vi "SGDA-Initialize Hardware.vi"(0 "Start PXI Server":bool=TRUE, 7 "TDT-Device Config":T1, 11 "error in (no error)":errorcluster) -> (8 "Hardware":T5, 15 "error out":errorcluster)   [LabVIEW 2020]
uses:
  Type Defs/Hardware Destination.ctl
  TDT VIs/Typedefs/TDT-Device Config.ctl
  TDT VIs/Typedefs/TDT-Output source.ctl
  TDT VIs/Typedefs/TDT-Device ID.ctl
  TDT VIs/Typedefs/TDT-Input source.ctl
  SGDA-Globals.vi
  <resource>/objmgr/daqmx.rc
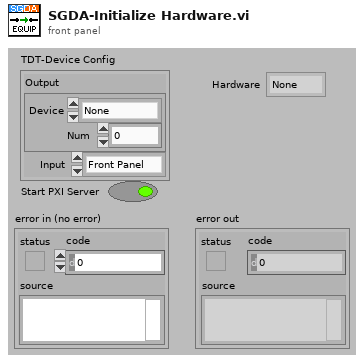
[diagram p1: front panel]
types:
  T1 = typedef "TDT-Device Config.ctl" = cluster{"Output":T2, "Input":T4}
  T2 = typedef "TDT-Output source.ctl" = cluster{"Device":T3, "Num":i32}
  T3 = typedef "TDT-Device ID.ctl" = enum16{"None", "PA5", "RP2", "RL2", "RA16", "RV8", "RX5", "RX6", "RX7", "RX8", "RZ2", "RZ5", "RZ6"}
  T4 = typedef "TDT-Input source.ctl" = enum16{"Front Panel", "RA4LI", "RA16LI"}
  T5 = typedef "Hardware Destination.ctl" = enum16{"None", "PXI", "TDT", "NI", "TDTSIM"}
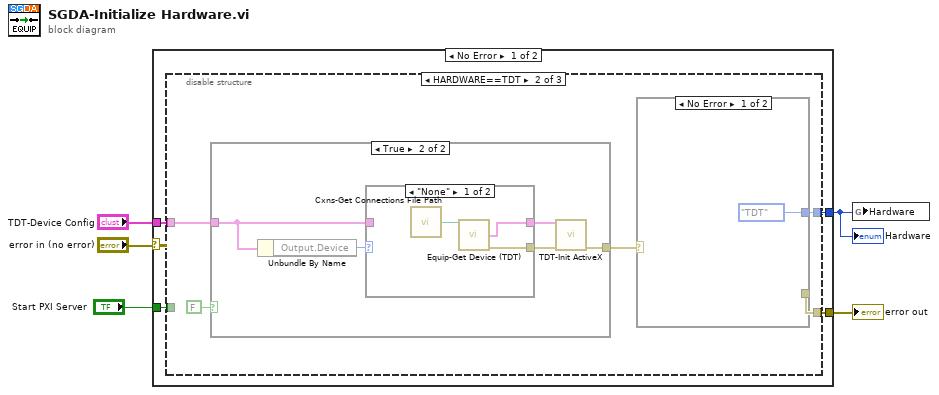
[diagram p0: block diagram]
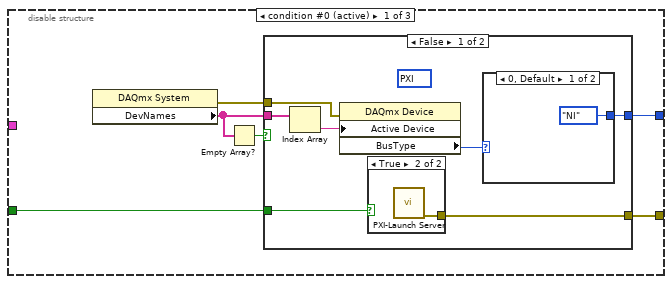
[diagram p2: hidden frame]
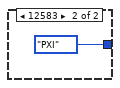
[diagram p4: hidden frame]
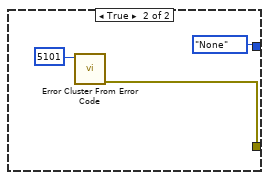
[diagram p5: hidden frame]
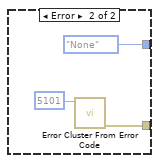
[diagram p8: hidden frame]
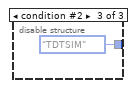
[diagram p9: hidden frame]
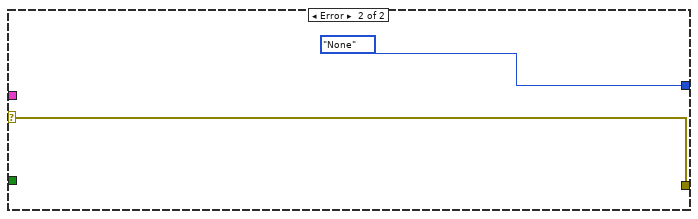
[diagram p10: hidden frame]
diagram:
  n1 = case shown="No Error" "error in (no error)" {
    selector: "error in (no error)" -> [_ w49]
    tunnel: [w9 w49] -> w4
    tunnel: [w8 Hardware_Destination."None" ("Hardware")] -> w3
    tunnel: "TDT-Device Config" -> [w7 _]
    tunnel: "Start PXI Server" -> [w6 _]
    frame No Error {
      n2 = disable-structure shown="HARDWARE==TDT" {
        disable-tunnel: [w15 w32 _] -> w9
        disable-tunnel: [w14 w31 Hardware_Destination."TDTSIM" ("Hardware")] -> w8
        disable-tunnel: w7 -> [_ w30 _]
        disable-tunnel: w6 -> [w13 _ _]
        frame condition #0 (active) {
          n3 = property class="DAQmx System"() -> (error out=w10:errorcluster, "DevNames"=w11:tag[])  [unwired: 2 in, 1 out]
          n4 = Empty Array?(array=w11) -> (empty?=w12:bool)
          n5 = case shown="False" w12 {
            tunnel: [w22 w27] -> w15
            tunnel: [w21 Hardware_Destination."None" ("Hardware")] -> w14
            tunnel: w11 -> [w20 _]
            tunnel: w10 -> [w18 _]
            tunnel: w13 -> [w16 _]
            frame False {
              (unwired) 12583 items=["PCI"=12582, "PCIe"=13612, "PXI"=12583, "PXIe"=14706, "SCXI"=12584, "SCC"=14707, "PCCard"=12585, "USB"=12586, "CompactDAQ"=14637, "TCP/IP"=14828, "Unknown"=12588, "SwitchBlock"=15870] ("BusType")
              n6 = Index Array(array=w20) -> (element=w19:tag)  [unwired: 1 in]
              n7 = property class="DAQmx Device"(error in=w18, "Active Device"=w19) -> ("BusType"=w17:i32)  [unwired: 1 in, 2 out]
              n8 = case shown="True" w16 {
                tunnel: [_ w23] -> w22
                frame False {
                }
                frame True {
                  n9 = call "PXI-Launch Server.vi"() -> ("error out"=w23:errorcluster)  [unwired: 10 in, 1 out]
                }
              }
              n10 = case shown="0, Default" w17 {
                tunnel: [Hardware_Destination."NI" ("Hardware") Hardware_Destination."PXI" ("Hardware")] -> w21
                frame 0, Default {
                }
                frame 12583 {
                }
              }
            }
            frame True {
              n11 = call <vilib>:"Error Cluster From Error Code.vi"("error code (0)"=5101) -> ("error out"=w27:errorcluster)  [unwired: 8 in]
            }
          }
        }
        frame condition #1 {
          n12 = case shown="True" FALSE {
            tunnel: [_ w38] -> w33
            tunnel: w30 -> [_ w36]
            frame False {
            }
            frame True {
              n13 = Unbundle By Name(w36) -> ("Output.Device"=w37:T3)
              n14 = case shown="\"None\"" w37 {
                tunnel: w36 -> [_ w42]
                tunnel: [w40 w42] -> w35
                tunnel: [w39 _] -> w34
                frame "None" {
                  n15 = call "Cxns-Get Connections File Path.vi"() -> ("Path Out"=w41:path)  [unwired: 1 in]
                  n16 = call "Equip-Get Device (TDT).vi"("Path In"=w41) -> ("TDT-Device Config"=w40:T1, "error out"=w39:errorcluster)  [unwired: 12 in, 1 out]
                }
                frame "PA5", Default {
                }
              }
              n17 = call "TDT-Init ActiveX.vi"("TDT-Device Config"=w35, "error in (no error)"=w34) -> ("error out"=w38:errorcluster)  [unwired: 10 in, 3 out]
            }
          }
          n18 = case shown="No Error" w33 {
            tunnel: [_ w46] -> w32
            tunnel: [Hardware_Destination."TDT" ("Hardware") Hardware_Destination."None" ("Hardware")] -> w31
            frame No Error {
            }
            frame Error {
              n19 = call <vilib>:"Error Cluster From Error Code.vi"("error code (0)"=5101) -> ("error out"=w46:errorcluster)  [unwired: 8 in]
            }
          }
        }
        frame condition #2 {
        }
      }
    }
    frame Error {
    }
  }
  "error out" <- w4
  "Hardware" <- w3
  n20 = global write "SGDA-Globals.vi" "Hardware"(w3) -> ()
